vi "Get AccelGyro constants (MCU EEPROM).vi"(0 "VISA resource name in":refnum<visa-resource-name>, 3 "Error In":errorcluster) -> (7 "VISA resource name out":refnum<visa-resource-name>, 8 "AccelGyro constants":T1={"gyrRange"=125.0, "accRange"=2.0, "gx offset"=0.0, "gy offset"=0.0, "gz offset"=0.0, "ax offset"=0.0, "ay offset"=0.0, "az offset"=0.0, "axyz scale"=1.0}, 9 "ACK":bool, 10 "Error out":errorcluster)   [LabVIEW 2015]
uses:
  Ctls/AccelGyro constants.ctl
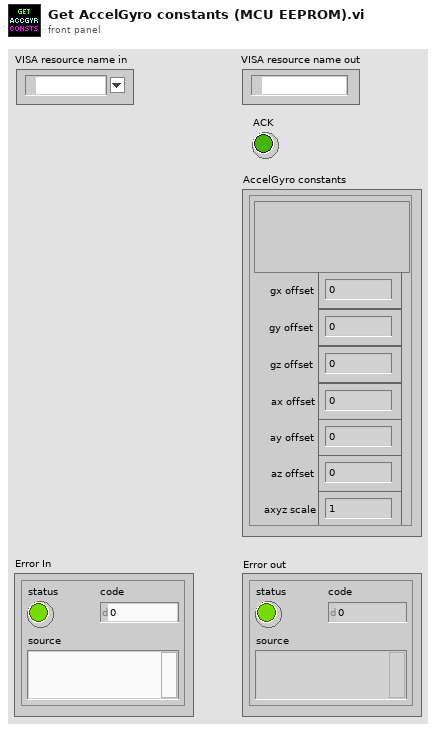
[diagram p1: front panel]
types:
  T1 = typedef "AccelGyro constants.ctl" = cluster{"gyrRange":sgl, "accRange":sgl, "gx offset":sgl, "gy offset":sgl, "gz offset":sgl, "ax offset":sgl, "ay offset":sgl, "az offset":sgl, "axyz scale":sgl}
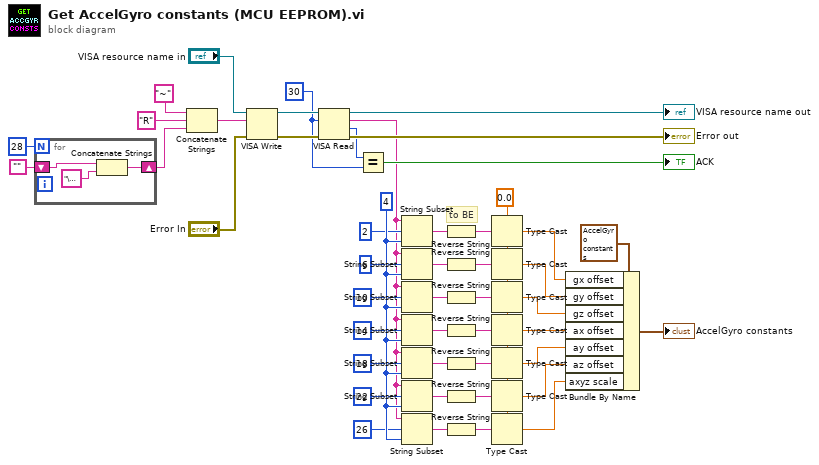
[diagram p0: block diagram]
diagram:
  w30 = 4 ("length (rest)")
  w31 = sgl 0.0
  w38 = u32 30 ("byte count")
  # "to BE"
  n1 = for {
    N: 28 -> [_]
    shift-right: [w50] -> w34
    shift-left: "" -> [w49]
    n2 = Concatenate Strings(w49, "\u0000") -> (w50:string)
  }
  n3 = Concatenate Strings("~" ("string"), "R" ("string"), w34) -> (w45:string)
  n4 = VISA Write(VISA resource name="VISA resource name in", write buffer=w45, error in (no error)="Error In") -> (VISA resource name out=w47:refnum<visa-resource-name>, error out=w46:errorcluster)  [unwired: 1 out]
  n5 = VISA Read(VISA resource name=w47, byte count=w38, error in (no error)=w46) -> (VISA resource name out=→"VISA resource name out":refnum<visa-resource-name>, read buffer=w15:string, return count=w39:u32, error out=→"Error out":errorcluster)
  n6 = Equal?(x=w39, y=w38) -> (x = y?=→"ACK":bool)
  n7 = String Subset(string=w15, offset (0)=2 ("length (rest)"), length (rest)=w30) -> (substring=w6:string)
  n8 = String Subset(string=w15, offset (0)=6 ("length (rest)"), length (rest)=w30) -> (substring=w5:string)
  n9 = String Subset(string=w15, offset (0)=10 ("length (rest)"), length (rest)=w30) -> (substring=w4:string)
  n10 = String Subset(string=w15, offset (0)=14 ("length (rest)"), length (rest)=w30) -> (substring=w3:string)
  n11 = String Subset(string=w15, offset (0)=18 ("length (rest)"), length (rest)=w30) -> (substring=w2:string)
  n12 = String Subset(string=w15, offset (0)=22 ("length (rest)"), length (rest)=w30) -> (substring=w1:string)
  n13 = String Subset(string=w15, offset (0)=26 ("length (rest)"), length (rest)=w30) -> (substring=w14:string)
  n14 = Reverse String(1:w6) -> (0:w7:string)
  n15 = Reverse String(1:w5) -> (0:w8:string)
  n16 = Reverse String(1:w4) -> (0:w9:string)
  n17 = Reverse String(1:w3) -> (0:w10:string)
  n18 = Reverse String(1:w2) -> (0:w11:string)
  n19 = Reverse String(1:w1) -> (0:w12:string)
  n20 = Reverse String(1:w14) -> (0:w13:string)
  n21 = Type Cast(type=w31, x=w7) -> (*(type *) &x=w17:sgl)
  n22 = Type Cast(type=w31, x=w8) -> (*(type *) &x=w18:sgl)
  n23 = Type Cast(type=w31, x=w9) -> (*(type *) &x=w19:sgl)
  n24 = Type Cast(type=w31, x=w10) -> (*(type *) &x=w20:sgl)
  n25 = Type Cast(type=w31, x=w11) -> (*(type *) &x=w21:sgl)
  n26 = Type Cast(type=w31, x=w12) -> (*(type *) &x=w32:sgl)
  n27 = Type Cast(type=w31, x=w13) -> (*(type *) &x=w33:sgl)
  n28 = Bundle By Name(cluster=T1 {"gyrRange"=0.0, "accRange"=0.0, "gx offset"=0.0, "gy offset"=0.0, "gz offset"=0.0, "ax offset"=0.0, "ay offset"=0.0, "az offset"=0.0, "axyz scale"=1.0} ("AccelGyro constants"), "gx offset"=w17, "gy offset"=w18, "gz offset"=w19, "ax offset"=w20, "ay offset"=w21, "az offset"=w32, "axyz scale"=w33) -> (→"AccelGyro constants":T1)
